vi "Add Buffer Channels.vi"(1 "byte order":T1, 4 "channels":T2[](array[typedef]) {"string offset" format="%d bytes"}, 5 "engine (T) / string (F)":bool, 6 "Decimation":u64, 7 "Transfer Group Status":refnum<class "Status.lvclass">, 8 "error in (no error)":errorcluster, 9 "Buffer":refnum<class "Buffer.lvclass">, 10 "parent tag":string, 11 "Application Data In":T5) -> (0 "error out":errorcluster, 3 "Application Data out":T5)   [LabVIEW 2017, in "DSF Core.lvlib"]
uses:
  DSF Core.lvlib
  Main VI/Application Data.ctl
  LabVIEW-Memory/Source/Classes/Pointer/Pointer.lvclass
  Classes/Framework/Framework.lvclass
  Buffer Reader/Buffer Data.ctl
  Classes/Buffer/Buffer.lvclass
  C:/Git/DSF/LabVIEW-Memory/Source/Classes/Pointer/Pointer.lvclass
  Classes/Transfer Group Status/Status.lvclass
  Typedefs/DSF Data Type.ctl
  Typedefs/DSF Engine Channel Configuration.ctl
  Typedefs/DSF Settings Info.ctl
  Typedefs/DSF Byte Order.ctl
  Typedefs/DSF Engine Framework Configuration.ctl
  Typedefs/DSF Engine Plugin Configuration.ctl
  Typedefs/DSF Timing Info.ctl
  Typedefs/DSF Engine Plugin Thread Configuration.ctl
  Typedefs/DSF Engine Transfer Group Configuration.ctl
  Typedefs/DSF Direction.ctl
  Typedefs/DSF Engine Transfer Configuration.ctl
  Typedefs/DSF Timeout Behavior.ctl
  ID to Tree Items/Tree Item Type.ctl
  Classes/Buffer/Get Buffer Size.vi
  LabVIEW-Memory/Source/Classes/Pointer/Get Size.vi
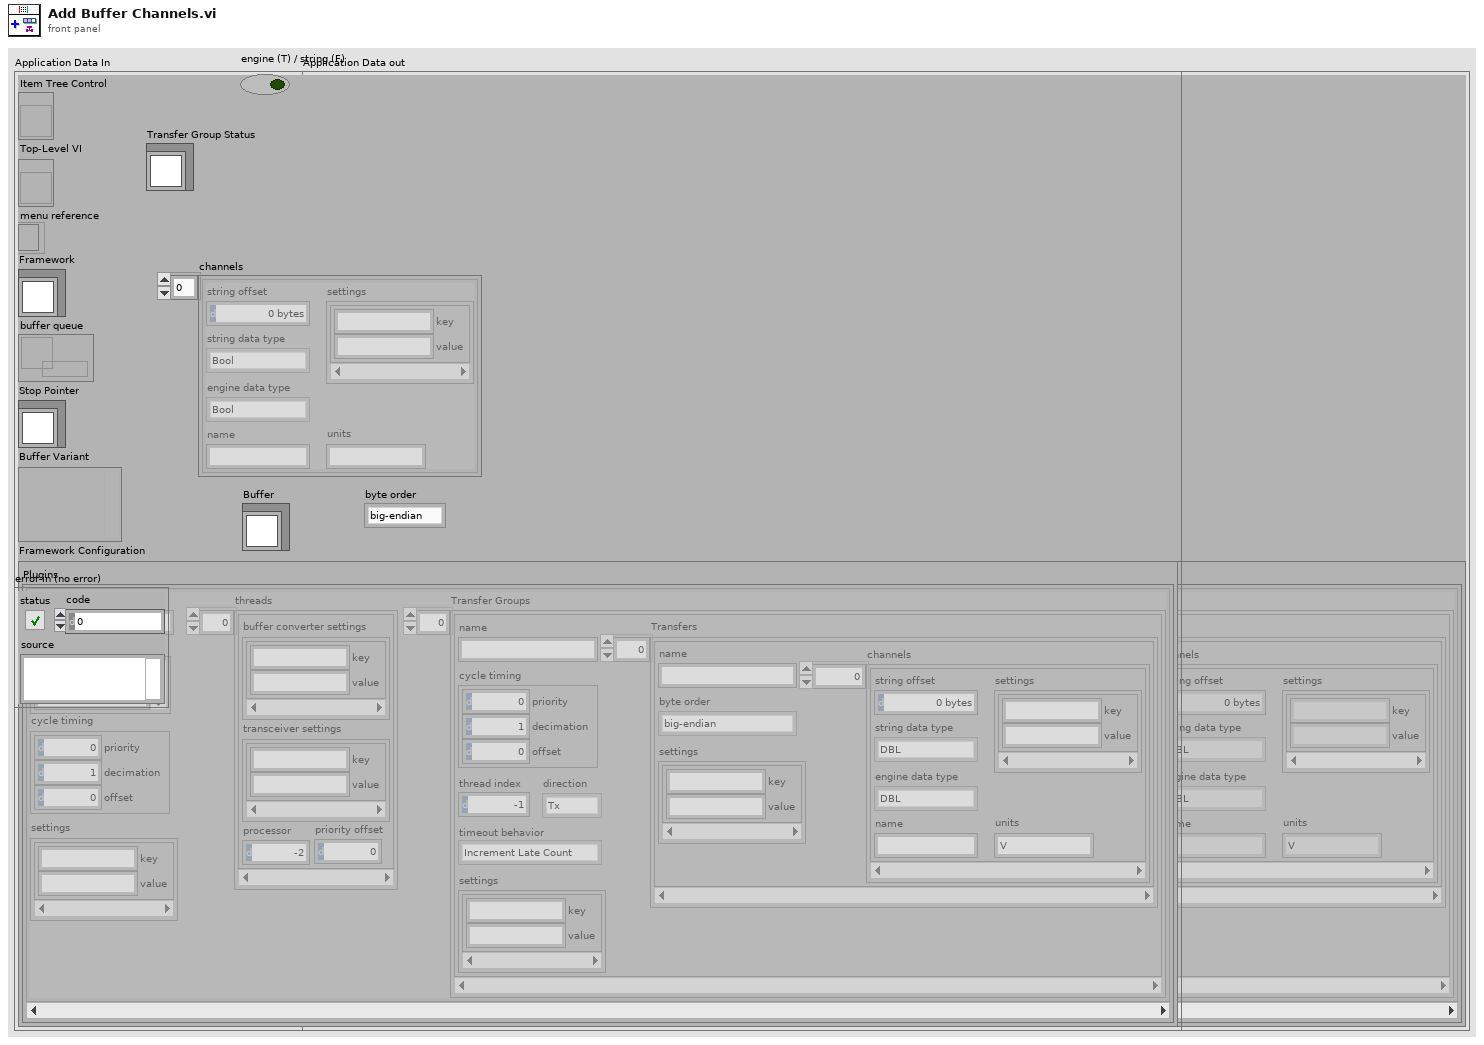
[diagram p1: front panel]
types:
  T1 = typedef "DSF Core.lvlib/DSF Byte Order.ctl" = enum8{"big-endian", "little-endian"}
  T2 = typedef "DSF Core.lvlib/DSF Engine Channel Configuration.ctl" = cluster{"string offset":u64, "string data type":T3, "engine data type":T3, "name":string, "settings":T4, "units":string}
  T3 = typedef "DSF Core.lvlib/DSF Data Type.ctl" = enum8{"Bool", "SGL", "DBL", "I8", "I16", "I32", "I64", "U8", "U16", "U32", "U64"}
  T4 = typedef "DSF Core.lvlib/DSF Settings Info.ctl" = cluster{"key":string, "value":string}[]
  T5 = typedef "DSF Core.lvlib/Application Data.ctl" = cluster{"Item Tree Control":refnum<vi>, "Top-Level VI":refnum<vi>, "menu reference":refnum<k9>, "Framework":refnum<class "Framework.lvclass">, "buffer queue":refnum<queue>, "Stop Pointer":refnum<class "Pointer.lvclass">, "Buffer Variant":variant, "Framework Configuration":T6}
  T6 = typedef "DSF Core.lvlib/DSF Engine Framework Configuration.ctl" = cluster{"Plugins":T7[]}
  T7 = typedef "DSF Core.lvlib/DSF Engine Plugin Configuration.ctl" = cluster{"name":string, "components":string[], "cycle timing":T8, "threads":T9[], "Transfer Groups":T10[], "settings":T4}
  T8 = typedef "DSF Core.lvlib/DSF Timing Info.ctl" = cluster{"priority":u64, "decimation":u64, "offset":u64}
  T9 = typedef "DSF Core.lvlib/DSF Engine Plugin Thread Configuration.ctl" = cluster{"buffer converter settings":T4, "transceiver settings":T4, "processor":i32, "priority offset":i16}
  T10 = typedef "DSF Core.lvlib/DSF Engine Transfer Group Configuration.ctl" = cluster{"name":string, "direction":T11, "cycle timing":T8, "thread index":i32, "settings":T4, "Transfers":T12[], "timeout behavior":T13}
  T11 = typedef "DSF Core.lvlib/DSF Direction.ctl" = enum8{"Tx", "Rx"}
  T12 = typedef "DSF Core.lvlib/DSF Engine Transfer Configuration.ctl" = cluster{"name":string, "byte order":T1, "settings":T4, "channels":T2[]}
  T13 = typedef "DSF Core.lvlib/DSF Timeout Behavior.ctl" = enum8{"Increment Late Count", "Throw Error"}
  T14 = typedef "DSF Core.lvlib/Buffer Data.ctl" = cluster{"Buffer":refnum<class "Buffer.lvclass">, "Status":refnum<class "Status.lvclass">, "decimation":u64, "avg bandwidth":dbl, "data type":T3, "units":string, "channels":T2[], "channel":bool, "engine (T) / string (F)":bool, "byte order":T1}
  T15 = typedef "DSF Core.lvlib/Tree Item Type.ctl" = enum16{"Framework", "Plugin Group", "Plugin", "Group", "Transfer", "Buffer", "Channel"}
  T16 = typedef "DSF Core.lvlib/Tree Item.ctl" = cluster{"Left Cell String":string, "Child Text":string[], "Child Tag":string, "Glyph Index":i32}
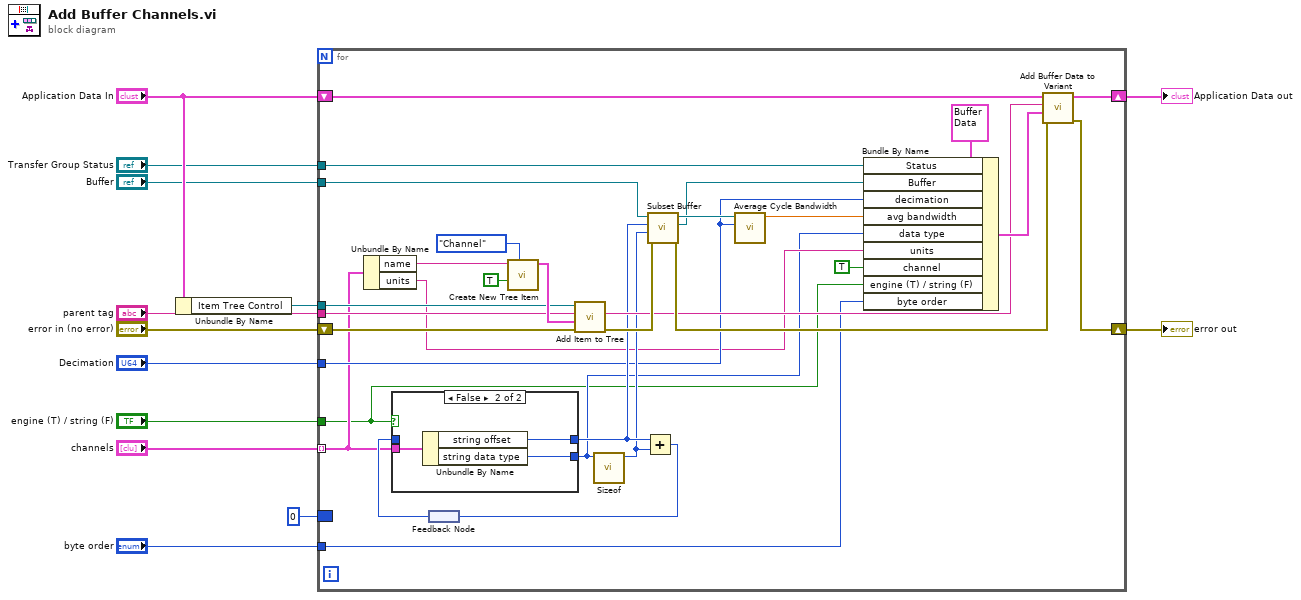
[diagram p0: block diagram]
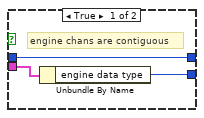
[diagram p2: hidden frame]
diagram:
  n1 = Unbundle By Name("Application Data In") -> ("Item Tree Control"=w9:refnum<vi>)
  n2 = for {
    tunnel: w9 -> [w35]
    tunnel: "parent tag" -> [w34]
    tunnel: "Transfer Group Status" -> [w33]
    tunnel: "Buffer" -> [w19]
    tunnel: "Decimation" -> [w22]
    shift-right: [w43] -> w12
    shift-left: "error in (no error)" -> [w40]
    shift-right: [w44] -> w13
    shift-left: "Application Data In" -> [w36]
    tunnel: "channels" -> [w21] mode=indexing
    tunnel: "engine (T) / string (F)" -> [w15]
    border: u64 0 -> [_]
    tunnel: "byte order" -> [w14]
    n3 = Unbundle By Name(w21) -> ("name"=w20:string, "units"=w18:string)
    n4 = feedback #1() -> (w29:u64)
    n5 = case shown="False" w15 {
      tunnel: w21 -> [w47 w50]
      tunnel: [w46 w49] -> w17
      tunnel: [w45 w48] -> w24
      tunnel: w29 -> [w45 _]
      frame True {
        # "engine chans are contiguous"
        n6 = Unbundle By Name(w47) -> ("engine data type"=w46:T3)
      }
      frame False {
        n7 = Unbundle By Name(w50) -> ("string offset"=w48:u64, "string data type"=w49:T3)
      }
    }
    n8 = call "Create New Tree Item.vi"("Item Type"=Tree_Item_Type."Channel", "found?"=TRUE, "Left Cell String"=w20) -> ("Item"=w37:T16)  [unwired: 7 in, 1 out]
    n9 = call "Add Item to Tree.vi"("error in (no error)"=w40, "Item"=w37, "parent tag"=w34, "TreeControl in"=w35) -> ("error out"=w27:errorcluster, "new item tag"=w25:string)  [unwired: 5 in, 1 out]
    n10 = call "Sizeof.vi"("data type"=w17) -> ("size in bytes"=w23:u64)  [unwired: 9 in, 1 out]
    n11 = Add(x=w24, y=w23) -> (x+y=w28:u64)
    n12 = feedback-in #1(w28) -> ()
    n13 = call "Subset Buffer.vi"("error in (no error)"=w27, "size"=w23, "offset"=w24, "Buffer in"=w19) -> ("error out"=w26:errorcluster, "subset Buffer"=w30:refnum<class "Buffer.lvclass">, "Buffer out"=w31:refnum<class "Buffer.lvclass">)  [unwired: 4 in, 1 out]
    n14 = call "Average Cycle Bandwidth.vi"("Decimation"=w22, "Buffer"=w31) -> ("avergage cycle bandwidth"=w32:dbl)  [unwired: 9 in]
    n15 = Bundle By Name(cluster=T14 {"Buffer"=refnum, "Status"=refnum, "decimation"=0, "avg bandwidth"=0.0, "data type"=enum."Bool", "units"="", "channels"=[], "channel"=FALSE, "engine (T) / string (F)"=FALSE, "byte order"=enum."little-endian"} ("Buffer data"), "Status"=w33, "Buffer"=w30, "decimation"=w22, "avg bandwidth"=w32, "data type"=w17, "units"=w18, "channel"=TRUE, "engine (T) / string (F)"=w15, "byte order"=w14) -> (w42:T14)
    n16 = call "Add Buffer Data to Variant.vi"("error in (no error)"=w26, "Buffer data"=w42, "tag"=w25, "Application Data In in"=w36) -> ("error out"=w43:errorcluster, "Application Data In out"=w44:T5)  [unwired: 6 in]
  }
  "error out" <- w12
  "Application Data out" <- w13
